vi "Calculate RF Cal Points.vi"(8 "error in (no error)":errorcluster, 10 "RF Calibration Parameters In":T4[](array[typedef]), 11 "New Sequence File Path":path) -> (0 "error out":errorcluster, 2 "Sweep Settings Data":T1[](array[typedef]) {"Sweep Points"."Frequency" format="%#_6p"})   [LabVIEW 2016]
uses:
  RFPM CLB Calibration/RFPM CLB Calibration UI.lvlibp/Actors/RFPM CLB Calibration UI/RFPM CLB Calibration UI/TypeDefs/Sweep Points.ctl
  RFPM CLB Calibration/RFPM CLB Calibration UI.lvlibp/Actors/RFPM CLB Calibration UI/RFPM CLB Calibration UI/RFPM CLB Calibration UI.lvclass
  niRFSTS Sequence Flow.lvclass
  RFPM CLB Calibration/RFPM CLB Calibration Process.lvlibp/RFPM CLB Calibration Process/TypeDefs/Sweep Type.ctl
  Typedefs/RF Calibration Parameters.ctl
  RFPM CLB Calibration/RFPM CLB Calibration UI.lvlibp/Actors/RFPM CLB Calibration UI/RFPM CLB Calibration UI/TypeDefs/Sweep Editor Data.ctl
  RFPM CLB Calibration/RFPM CLB Calibration UI.lvlibp/Actors/RFPM CLB Calibration Process/RFPM CLB Calibration Process/TypeDefs/Sweep Type.ctl
  RFPM CLB Calibration/RFPM CLB Calibration UI.lvlibp/Actors/RFPM CLB Calibration Process/RFPM CLB Calibration Process/RFPM CLB Calibration Process.lvclass
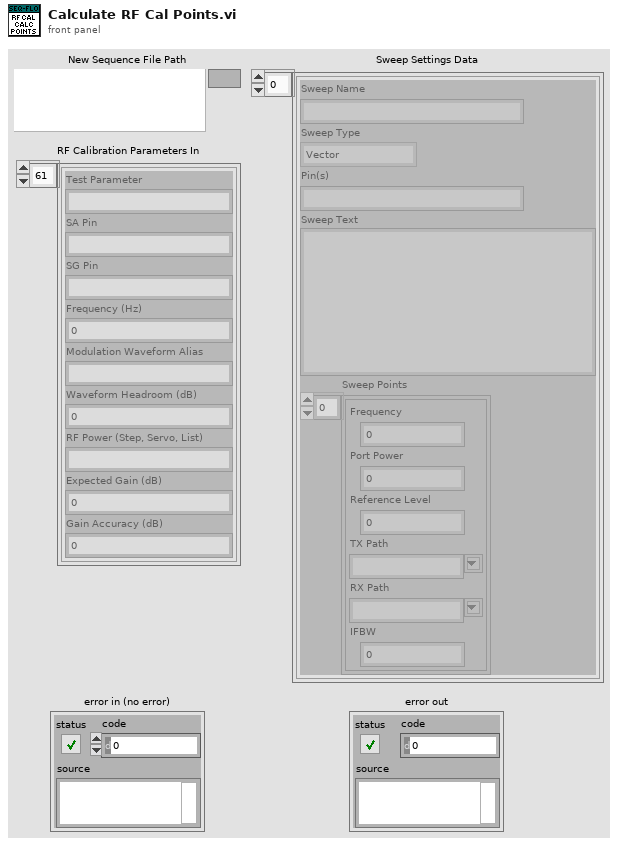
[diagram p1: front panel]
types:
  T1 = typedef "RFPM CLB Calibration UI.lvclass/Sweep Editor Data.ctl" = cluster{"Sweep Name":string, "Sweep Type":T2, "Pin(s)":string, "Sweep Text":string, "Sweep Points":T3[]}
  T2 = typedef "RFPM CLB Calibration UI.lvlibp/RFPM CLB Calibration Process.lvlib/RFPM CLB Calibration Process.lvclass/Sweep Type.ctl" = enum16{"Vector", "Source", "Receiver"}
  T3 = typedef "RFPM CLB Calibration UI.lvclass/Sweep Points.ctl" = cluster{"Frequency":dbl, "Port Power":dbl, "Reference Level":dbl, "TX Path":string, "RX Path":string, "IFBW":dbl}
  T4 = typedef "niRFSTS Sequence Flow.lvclass/RF Calibration Parameters.ctl" = cluster{"Test Parameter":string, "SA Pin":string, "SG Pin":string, "Frequency (Hz)":dbl, "Modulation Waveform Alias":string, "Waveform Headroom (dB)":dbl, "RF Power (Step, Servo, List)":string, "Expected Gain (dB)":dbl, "Gain Accuracy (dB)":dbl}
  T5 = typedef "RFPM CLB Calibration Process.lvlibp/RFPM CLB Calibration Process.lvclass/Sweep Type.ctl" = enum16{"Vector", "Source", "Receiver"}
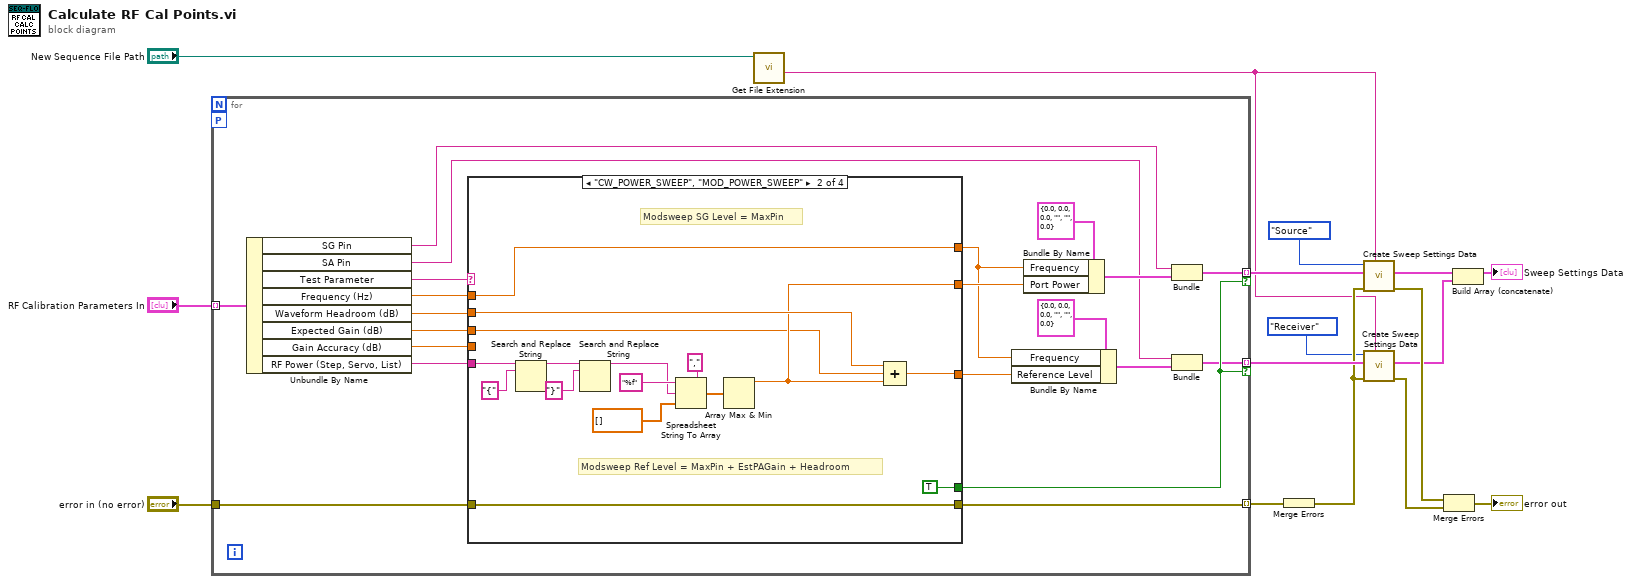
[diagram p0: block diagram]
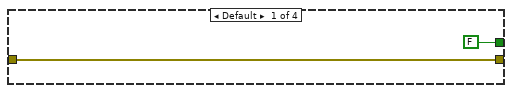
[diagram p2: hidden frame]
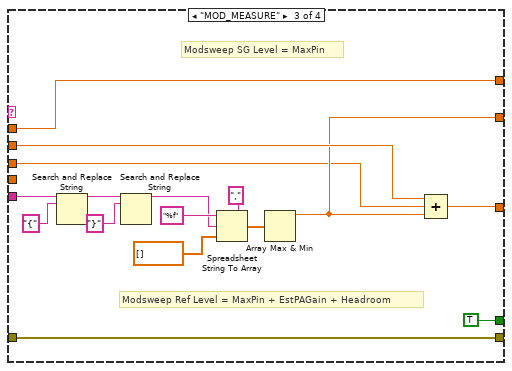
[diagram p3: hidden frame]
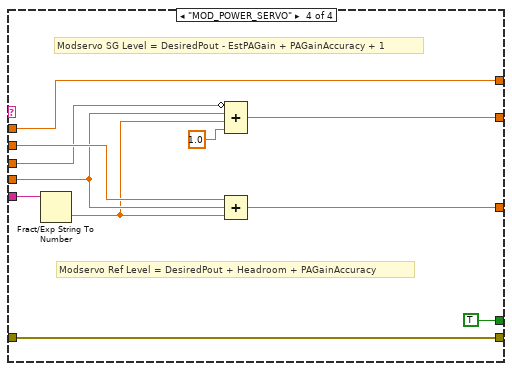
[diagram p4: hidden frame]
diagram:
  n1 = for {
    tunnel: "RF Calibration Parameters In" -> [w37] mode=indexing
    tunnel: "error in (no error)" -> [w34]
    tunnel: [w33] -> w14 mode=indexing
    tunnel: [w20] -> w13 mode=indexing if=w24
    tunnel: [w18] -> w12 mode=indexing if=w24
    workers-P: _ -> [_]
    n2 = Unbundle By Name(w37) -> ("SG Pin"=w22:string, "SA Pin"=w21:string, "Test Parameter"=w36:string, "Frequency (Hz)"=w35:dbl, "Waveform Headroom (dB)"=w32:dbl, "Expected Gain (dB)"=w17:dbl, "Gain Accuracy (dB)"=w31:dbl, "RF Power (Step, Servo, List)"=w30:string)
    n3 = case shown="\"CW_POWER_SWEEP\", \"MOD_POWER_SWEEP\"" w36 {
      tunnel: w35 -> [_ w52 w68 w73]
      tunnel: w34 -> [w39 w55 w71 w82]
      tunnel: [w39 w55 w71 w82] -> w33
      tunnel: w17 -> [_ w45 w61 w79]
      tunnel: w32 -> [_ w54 w70 w80]
      tunnel: w31 -> [_ _ _ w78]
      tunnel: w30 -> [_ w41 w57 w81]
      tunnel: [_ w46 w62 w75] -> w28
      tunnel: [_ w53 w69 w74] -> w25
      tunnel: [_ w52 w68 w73] -> w26
      tunnel: [FALSE TRUE TRUE TRUE] -> w24
      frame Default {
      }
      frame "CW_POWER_SWEEP", "MOD_POWER_SWEEP" {
        # "Modsweep Ref Level = MaxPin + EstPAGain + Headroom"
        # "Modsweep SG Level = MaxPin"
        n4 = Search and Replace String(input string=w41, search string="{") -> (result string=w43:string)  [unwired: 6 in, 3 out]
        n5 = Search and Replace String(input string=w43, search string="}") -> (result string=w40:string)  [unwired: 6 in, 3 out]
        n6 = Spreadsheet String To Array(delimiter (Tab)=",", format string="%f", spreadsheet string=w40, array type (2D Dbl)=dbl[] []) -> (array=w47:dbl[])
        n7 = Array Max & Min(array=w47) -> (max value=w46:dbl)  [unwired: 3 out]
        n8 = Compound Arithmetic op=ADD(w54, w45, w46) -> (w53:dbl)
      }
      frame "MOD_MEASURE" {
        # "Modsweep Ref Level = MaxPin + EstPAGain + Headroom"
        # "Modsweep SG Level = MaxPin"
        n9 = Search and Replace String(input string=w57, search string="{") -> (result string=w59:string)  [unwired: 6 in, 3 out]
        n10 = Search and Replace String(input string=w59, search string="}") -> (result string=w56:string)  [unwired: 6 in, 3 out]
        n11 = Spreadsheet String To Array(delimiter (Tab)=",", format string="%f", spreadsheet string=w56, array type (2D Dbl)=dbl[] []) -> (array=w63:dbl[])
        n12 = Array Max & Min(array=w63) -> (max value=w62:dbl)  [unwired: 3 out]
        n13 = Compound Arithmetic op=ADD(w70, w61, w62) -> (w69:dbl)
      }
      frame "MOD_POWER_SERVO" {
        # "Modservo Ref Level = DesiredPout + Headroom + PAGainAccuracy"
        # "Modservo SG Level = DesiredPout - EstPAGain + PAGainAccuracy + 1"
        n14 = Fract/Exp String To Number(string=w81) -> (number=w77:dbl)  [unwired: 3 in, 1 out]
        n15 = Compound Arithmetic op=ADD(invert w79, w78, w77, 1.0 ("value")) -> (w75:dbl)
        n16 = Compound Arithmetic op=ADD(w80, w78, w77) -> (w74:dbl)
      }
    }
    n17 = Bundle By Name(cluster=T3 {"Frequency"=0.0, "Port Power"=0.0, "Reference Level"=0.0, "TX Path"="", "RX Path"="", "IFBW"=0.0} ("Sweep Point"), "Frequency"=w26, "Reference Level"=w25) -> (w19:T3)
    n18 = Bundle By Name(cluster=T3 {"Frequency"=0.0, "Port Power"=0.0, "Reference Level"=0.0, "TX Path"="", "RX Path"="", "IFBW"=0.0} ("Sweep Point"), "Frequency"=w26, "Port Power"=w28) -> (w23:T3)
    n19 = Bundle("SG Pin"=w22, "Sweep Point"=w23) -> (w20:cluster{"SG Pin":string, "Sweep Point":T3})  [unwired: 1 in]
    n20 = Bundle("SA Pin"=w21, "Sweep Point"=w19) -> (w18:cluster{"SA Pin":string, "Sweep Point":T3})  [unwired: 1 in]
  }
  n21 = call <vilib>:"Get File Extension.vi"("file"="New Sequence File Path") -> ("filename without extension"=w2:string)  [unwired: 6 in, 4 out]
  n22 = Merge Errors(w14) -> (w7:errorcluster)
  n23 = call "Create Sweep Settings Data.vi"("DUT Name"=w2, "error in (no error)"=w7, "Sweep Points"=w13, "Sweep Type"=Sweep_Type."Source") -> ("error out"=w10:errorcluster, "Sweep Settings Data"=w6:T1[])  [unwired: 6 in]
  n24 = call "Create Sweep Settings Data.vi"("DUT Name"=w2, "error in (no error)"=w7, "Sweep Points"=w12, "Sweep Type"=Sweep_Type."Receiver") -> ("error out"=w9:errorcluster, "Sweep Settings Data"=w5:T1[])  [unwired: 6 in]
  n25 = Merge Errors(w10, w9) -> (→"error out":errorcluster)
  n26 = Build Array (concatenate)(w6, w5) -> (→"Sweep Settings Data":T1[])
